vi "global.vi"() -> ()   [LabVIEW 2011]
uses:
  Hardware Control/OSC/SubVIs/controls/sampling_rate.ctl
  Hardware Control/OSC/SubVIs/controls/scale.ctl
panel:
  in  "TRIG inhibit off":dbl=9.999999999999999e-05 min=0.0 max=999.999999999995 format="%.1p"
  in  "TRIG mol delay":dbl=9.999999999999999e-05 min=0.0 max=999.999999999995 format="%.1p"
  in  "EXP chirp end":dbl=5000.0
  in  "EXP Meas Period":dbl=10.0 min=1.0 step=1.0
  in  "PSG Amplitude 2":dbl=10000000000.0 format="%#_6p"
  in  "PSG Amplitude 1":dbl=10000000000.0 format="%#_6p"
  in  "PSG steps":i32=10
  in  "PSG step size":dbl=2000000000.0 format="%#_6p"
  in  "PSG freq offset":dbl=2000000000.0 format="%#_6p"
  in  "PSG start freq":dbl=10000000000.0 format="%#_6p"
  in  "EXP Meas Cycles":i32=5000
  in  "TRIG burst enabled":bool=TRUE caption="Burst"
  in  "TRIG delay duration":dbl=4.6625e-05 format="%#_6p"
  in  "TRIG duration":dbl[](array[numeric])=[5.65e-06, 4.9999999999999996e-06, 4e-05, 4.9999999999999996e-06] min=0.0 format="%.3p"
  in  "TRIG start time":dbl[](array[numeric])=[0.0, 1.1e-06, 6.6e-06, 6.4e-06] format="%.3p"
  in  "TRIG burst period":dbl=4.9999999999999975e-05 format="%#_6p"
  in  "TRIG burst count":i32=1
  in  "OSC resolution":ext=24999.999999999999998 format="%#_6p"
  in  "OSC sample points":i32=200000
  in  "OSC hor scale":T1=4e-06 items=["400ns/div"=4e-07, "1µs/div"=1e-06, "2µs/div"=2e-06, "4µs/div"=4e-06, "10µs/div"=1e-05, "20µs/div"=2e-05]
  in  "OSC sample rate":T2=5000000000.0 items=["20 GHz (50ps/sample)", "10 GHz (100ps/sample)", "5.0 GHz (200ps/sample)", "2.5 GHz (400ps/sample)", "1.25 GHz (0.8ns/sample)", "0.5 GHz (2ns/sample)"]
  in  "TRIG BG cycle":dbl=100.0 min=0.0 max=999.999999999995 format="%.1p"
  # "Experiment Settings"
  # "OSC Settings"
  # "PSG Settings"
  # "TRIG2 Settings"
  # "TRIG1 Settings"
  # "all values are stored in standard SI units (seconds, hz, etc... no micro seconds or kHz or anything!)"
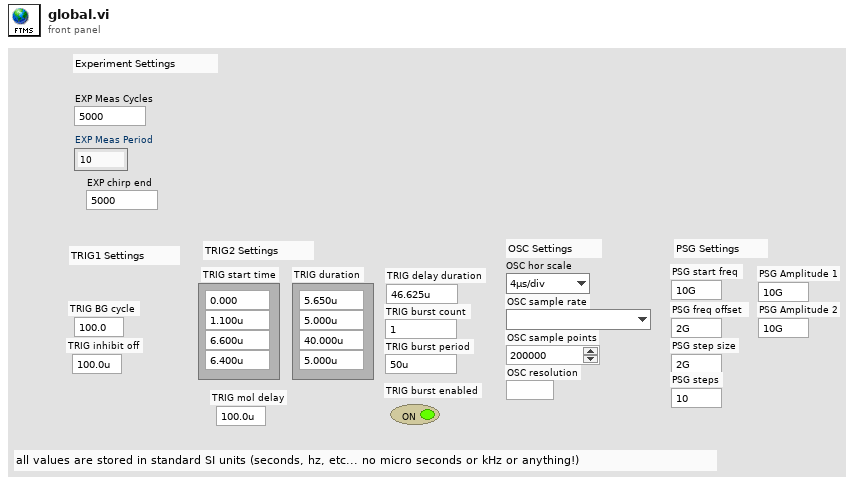
[diagram p1: front panel]
types:
  T1 = typedef "scale.ctl" = dbl
  T2 = typedef "sampling_rate.ctl" = ext
diagram:
